vi "MM DAQ.vi"(8 "error in":errorcluster, 10 "DAQ dt":i32, 11 "Multimeter in":refnum<class "Multimeter.lvclass">) -> (0 "error out":errorcluster, 2 "Data":dbl[](array[numeric]), 3 "Multimeter out":refnum<class "Multimeter.lvclass">)   [LabVIEW 2011]
uses:
  Modules/Hardware/Multimeter/Multimeter.lvclass
  <vilib>/Platform/TimedLoop/XDataNode/timing_clust.ctl
  <vilib>/Platform/TimedLoop/XDataNode/nitl_modes.ctl
  <vilib>/Platform/TimedLoop/XDataNode/wakeup.ctl
  Controls/User Interface Action.ctl
  <vilib>/Platform/TimedLoop/XDataNode/XDataNode.xnode
  <vilib>/Platform/TimedLoop/XDataNode/XDNodeRunTimeDep.lvlib
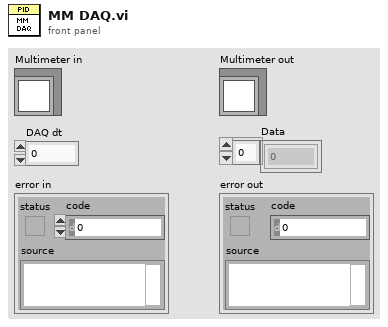
[diagram p1: front panel]
types:
  T1 = typedef "User Interface Action.ctl" = enum16{"Initialize", "Data Acquisition Disable", "Data View Disable", "Sample Set", "Sample Set 2D Data", "Sample Set x0 & dx", "Sample Add", "Sample Set Cursor", "Sample Set Offset & Multiplier", "Sample Set Axis Labels", "Sample Parameters Disabled", "Sample Parameters Update", "Run Update", "Run Set Offset & Multiplier", "Run Set Axis Labels", "Run Set Cursor", "Run Set Disabled", "Run Parameters Update", "Run Parameters Disabled", "Run Number Set", "Run Number Set Range", "Run Number Set Disabled", "Sample Number Set", "Sample Number Set Range", "Notes Set Value", "Update Plot", "Set Plot Parameters", "Update Concentration Plot", "Time Set", "Clear DAQ Display", "Clear Analysis Display", "Status Bar Set", "Progress Bar Set", "Display Mode Set", "Experiment Type Set", "Analysis Plot Average Set", "Stop"}
  T2 = typedef "XDNodeRunTimeDep.lvlib/timing_clust.ctl" = cluster{"Expected End [f-1]":u64, "Actual End [f-1]":u64, "Finished Late? [f-1]":bool, "Expected End [i-1]":u64, "Actual End [i-1]":u64, "Finished Late? [i-1]":bool, "Expected Start [i]":u64, "Actual Start [i]":u64, "Expected Start [f]":u64, "Actual Start [f]":u64, "Source Name":string, "Structure Name":string, "Period":i64, "Deadline":i64, "Offset":i64, "Start":i64, "Priority":i32, "Timeout":i32, "Mode":T3, "Wakeup Reason":T4, "Error":errorcluster, "Source Type":string, "Secondary Source Type":string, "Global End Time":u64, "Global Start Time":u64, "Frame Duration":u64, "Iteration Duration":u64, "Assigned CPU":i32, "I/O Scan Engine Mode":u32}
  T3 = typedef "XDNodeRunTimeDep.lvlib/nitl_modes.ctl" = enum32{"No Change", "Process missed periods, maintain original phase", "Discard missed periods, maintain original phase", "Process missed periods, ignore original phase", "Discard missed periods, ignore original phase"}
  T4 = typedef "XDNodeRunTimeDep.lvlib/wakeup.ctl" = enum32{"Normal", "Aborted", "Asynchronous wakeup", "Timing source error", "Timed loop error", "Timeout"}
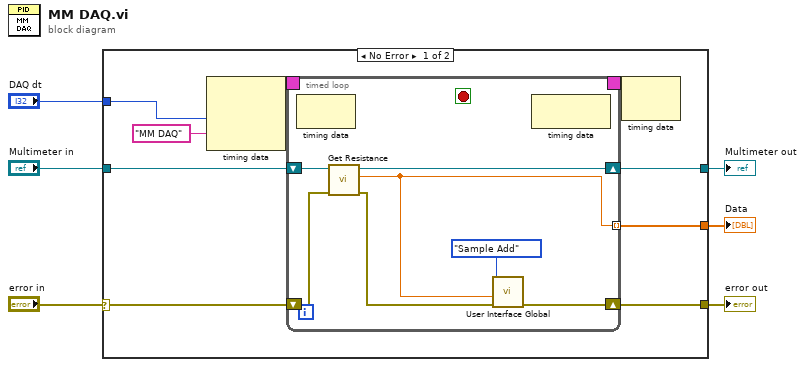
[diagram p0: block diagram]
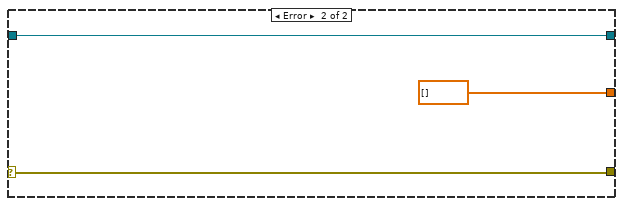
[diagram p2: hidden frame]
diagram:
  n1 = case shown="No Error" "error in" {
    selector: "error in" -> [w7 w30]
    tunnel: "DAQ dt" -> [w13 _]
    tunnel: "Multimeter in" -> [w11 w32]
    tunnel: [w10 w32] -> w4
    tunnel: [w9 w30] -> w3
    tunnel: [w8 dbl[] []] -> w2
    frame No Error {
      n2 = node-c288(w13, "MM DAQ" ("Structure Name")) -> (w15:T2)  [unwired: 1 in]
      n3 = timed-loop {
        timing: w15 -> [_]
        timing-out: [_] -> w14
        shift-right: [w18] -> w10
        shift-left: w11 -> [w22]
        shift-right: [w17] -> w9
        shift-left: w7 -> [w21]
        tunnel: [w16] -> w8 mode=indexing
        stop <- _ stop-if-true
        n4 = node-c288() -> ()  [unwired: 1 in, 1 out]
        n5 = call-dynamic "Get Resistance.vi"("error in (no error)"=w21, "Multimeter in"=w22) -> ("error out"=w19:errorcluster, "Resistance"=w16:dbl, "Multimeter out"=w18:refnum<class "Multimeter.lvclass">)  [unwired: 7 in]
        n6 = call "User Interface Global.vi"("error in"=w19, "data1"=w16, "action"=User_Interface_Action."Sample Add") -> ("error out"=w17:errorcluster)  [unwired: 8 in]
        n7 = node-c288() -> ()  [unwired: 1 in, 1 out]
      }
      n8 = node-c288(w14) -> ()  [unwired: 1 out]
    }
    frame Error {
    }
  }
  "error out" <- w3
  "Multimeter out" <- w4
  "Data" <- w2
